vi "Delta Tiime.get.vi"(8 "error in (no error)":errorcluster, 11 "midi-file-event in":refnum<class "midi-file-event.lvclass">) -> (0 "error out":errorcluster, 2 "Delta Tiime":u32, 3 "midi-file-event out":refnum<class "midi-file-event.lvclass">)   [LabVIEW 2020, in "midi-file-event.lvclass"]
uses:
  midi-file-event.lvclass
  midi-file-event.lvclass/midi-file-event.ctl
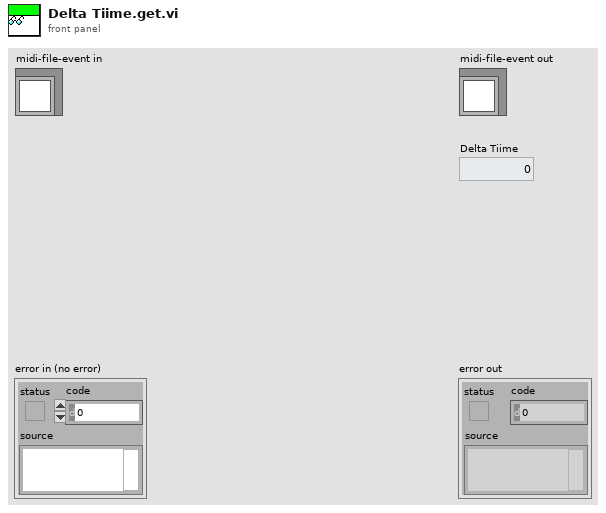
[diagram p1: front panel]
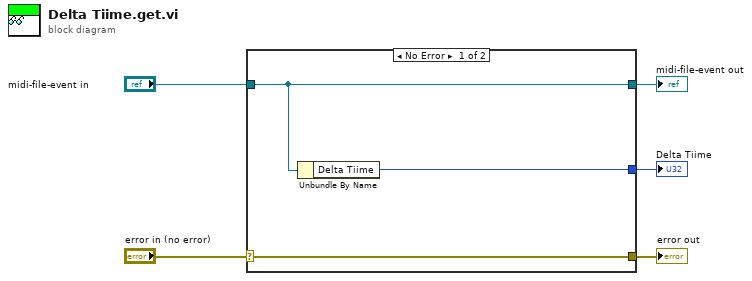
[diagram p0: block diagram]
diagram:
  n1 = case shown="No Error" "error in (no error)" {
    selector: "error in (no error)" -> [w8 w9]
    tunnel: [w8 w9] -> w4
    tunnel: [w7 w10] -> w2
    tunnel: "midi-file-event in" -> [w7 w10]
    tunnel: [w6 _] -> w1
    frame No Error {
      n2 = Unbundle By Name(w7) -> ("Delta Tiime"=w6:u32)
    }
    frame Error {
    }
  }
  "error out" <- w4
  "midi-file-event out" <- w2
  "Delta Tiime" <- w1
